vi "CRYUnFlatten End.vi"(7 "error in (no error)":errorcluster, 10 "Unflatten End setup":string) -> (0 "error out":errorcluster, 3 "Header of common":T2)   [LabVIEW 2013]
uses:
  Typedef Control/CRYHeader Cluster.ctl
  Typedef Control/CRYEnd Cluster.ctl
panel:
  out "End Cluster Step":T1
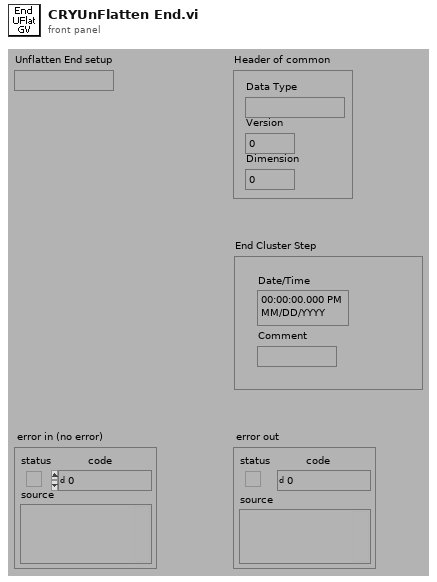
[diagram p1: front panel]
types:
  T1 = typedef "CRYEnd Cluster.ctl" = cluster{"Comment":string, "Date/Time":timestamp}
  T2 = typedef "CRYHeader Cluster.ctl" = cluster{"Data Type":string, "Version":u16, "Dimension":u8}
  T3 = cluster{"Comment":string, "seconds since 1Jan1904":timestamp}
  T4 = cluster{"unsigned byte array[0]":u8, "unsigned byte array[1]":u8, "unsigned byte array[2]":u8}
  T5 = cluster{"Unflatten End setup":string, u16, "unsigned byte array[2]":u8}
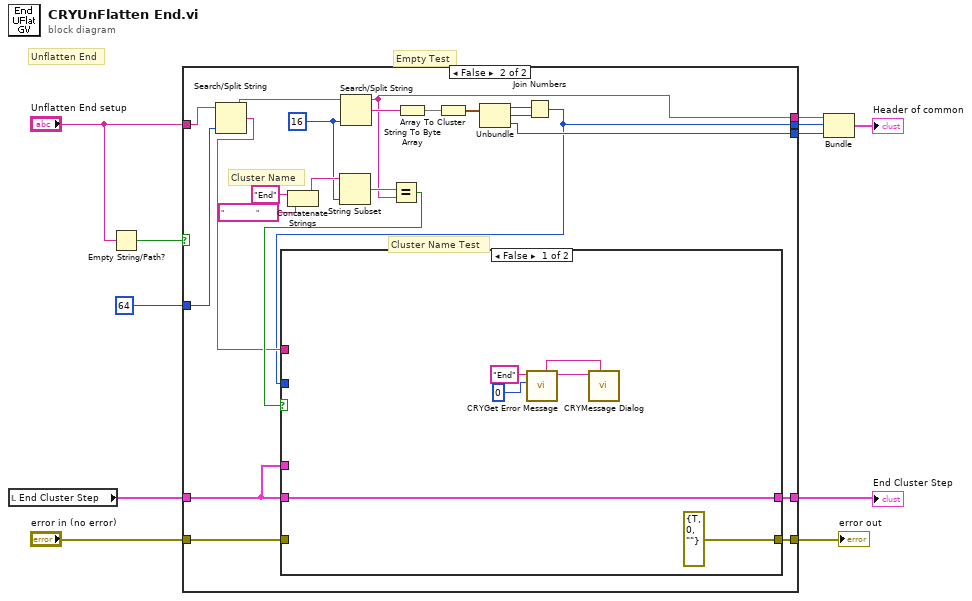
[diagram p0: block diagram]
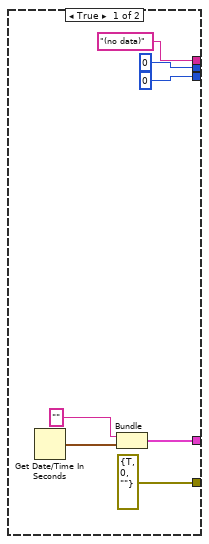
[diagram p2: hidden frame]
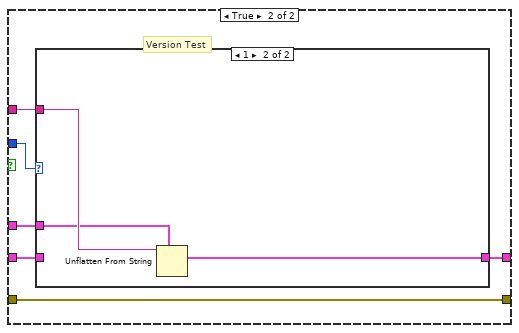
[diagram p3: hidden frame]
diagram:
  # "Empty Test"
  # "Unflatten End"
  n1 = local read "End Cluster Step"() -> (w2:T1)
  n2 = Empty String/Path?(string/path="Unflatten End setup") -> (empty?=w10:bool)
  n3 = case shown="False" w10 {
    tunnel: "Unflatten End setup" -> [_ w23]
    tunnel: 64 -> [_ w36]
    tunnel: [w12 w19] -> w1
    tunnel: [u16 0 w24] -> w7
    tunnel: [u8 0 w27] -> w6
    tunnel: ["(no data)" w26] -> w5
    tunnel: w2 -> [_ w22]
    tunnel: [errorcluster {"status"=TRUE, "code"=0, "source"=""} ("error in (no error)") w21] -> w4
    tunnel: "error in (no error)" -> [_ w20]
    frame True {
      n4 = Get Date/Time In Seconds() -> (seconds since 1Jan1904=w13:timestamp)
      n5 = Bundle("Comment"="", "seconds since 1Jan1904"=w13) -> (w12:T3)  [unwired: 1 out]
    }
    frame False {
      w34 = 16 ("length (rest)")
      # "Cluster Name Test"
      # "Cluster Name"
      n6 = Search/Split String(string=w23, offset (0)=w36) -> (substring before match=w35:string, match + rest of string=w25:string)  [unwired: 2 out]
      n7 = Concatenate Strings("End" ("string"), "                " ("string")) -> (w40:string)
      n8 = String Subset(string=w40, length (rest)=w34) -> (substring=w37:string)  [unwired: 1 out]
      n9 = Search/Split String(string=w35, offset (0)=w34) -> (substring before match=w26:string, match + rest of string=w33:string)  [unwired: 2 out]
      n10 = Equal?(x=w37, y=w26) -> (x = y?=w28:bool)
      n11 = String To Byte Array(string=w33) -> (unsigned byte array=w32:u8[])
      n12 = Array To Cluster(array=w32) -> (cluster=w31:T4)
      n13 = Unbundle(w31) -> ("unsigned byte array[0]"=w30:u8, "unsigned byte array[1]"=w29:u8, "unsigned byte array[2]"=w27:u8)
      n14 = Join Numbers(hi=w30, lo=w29) -> ((hi.lo)=w24:u16)
      n15 = case shown="False" w28 {
        tunnel: w25 -> [_ w49]
        tunnel: w24 -> [_ w51]
        tunnel: [w46 w50] -> w19
        tunnel: w22 -> [w46 w52]
        tunnel: w22 -> [_ w48]
        tunnel: [errorcluster {"status"=TRUE, "code"=0, "source"=""} ("error in (no error)") w47] -> w21
        tunnel: w20 -> [_ w47]
        frame False {
          n16 = call "CRYGet Error Message.vi"("Error No"=0, "Kind"="End") -> ("Message"=w42:string, "Window Title"=w41:string)  [unwired: 4 in, 4 out]
          n17 = call "CRYMessage Dialog.vi"("Window Title"=w41, "Message Content"=w42) -> ()  [unwired: 8 in, 2 out]
        }
        frame True {
          # "Version Test"
          n18 = case shown="1" w51 {
            tunnel: w52 -> [w53 _]
            tunnel: [w53 w55] -> w50
            tunnel: w49 -> [_ w56]
            tunnel: w48 -> [_ w54]
            frame 0, Default {
            }
            frame 1 {
              n19 = Unflatten From String(type=w54, binary string=w56) -> (value=w55:T1)  [unwired: 1 in, 4 out]
            }
          }
        }
      }
    }
  }
  "error out" <- w4
  "End Cluster Step" <- w1
  n20 = Bundle("Unflatten End setup"=w5, w7, "unsigned byte array[2]"=w6) -> (→"Header of common":T5)  [unwired: 1 out]
